vi "photo_encoder_new.vi"() -> ()   [LabVIEW 2014]
panel:
  in  "Brightness of Mark":dbl
  in  "Photo Value(placeholder for sensor data)":dbl
  out "Marks":i16
  # "This VI recognizes significant increases in brightness as \"marks\" and outputs the number of marks detected in the last second.\nKnown issues:  Does not reset M/s consistently, since all marks detected are handled with just one 10ms counter."
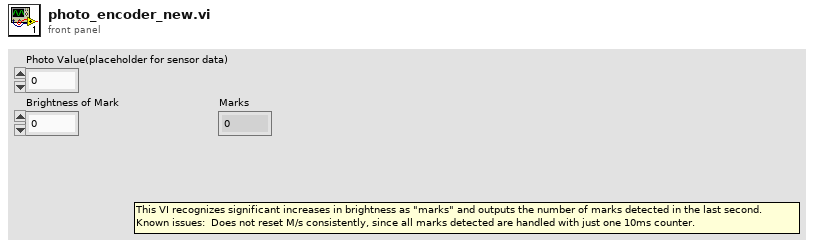
[diagram p1: front panel]
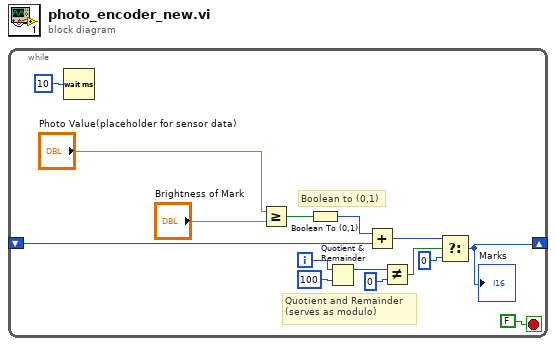
[diagram p0: block diagram]
diagram:
  n1 = while {
    shift-right: [w6] -> _
    shift-left: _ -> [w13]
    i -> [w9]
    stop <- FALSE stop-if-true
    # "Quotient and Remainder\n(serves as modulo)"
    # "Boolean to (0,1)"
    n2 = Wait (ms)(milliseconds to wait=u32 10) -> ()  [unwired: 1 out]
    n3 = Greater Or Equal?(x="Photo Value(placeholder for sensor data)", y="Brightness of Mark") -> (x >= y?=w1:bool)
    n4 = Boolean To (0,1)(Boolean=w1) -> (0, 1=w14:i16)
    n5 = Quotient & Remainder(x=w9, y=100) -> (x-y*floor(x/y)=w11:i32)  [unwired: 1 out]
    n6 = Add(x=w14, y=w13) -> (x+y=w7:i16)
    n7 = Not Equal?(x=w11, y=0) -> (x != y?=w12:bool)
    n8 = Select(t=w7, s=w12, f=i16 0) -> (s? t:f=w6:i16)
    "Marks" <- w6
  }
